vi "CmdExe.Text Log.vi"(7 "PrevLog":string, 8 "Rtn":i32, 9 "StdErr":string, 10 "StdOut":string, 11 "Cmd":string) -> (3 "CmdLog":string)   [LabVIEW 2019]
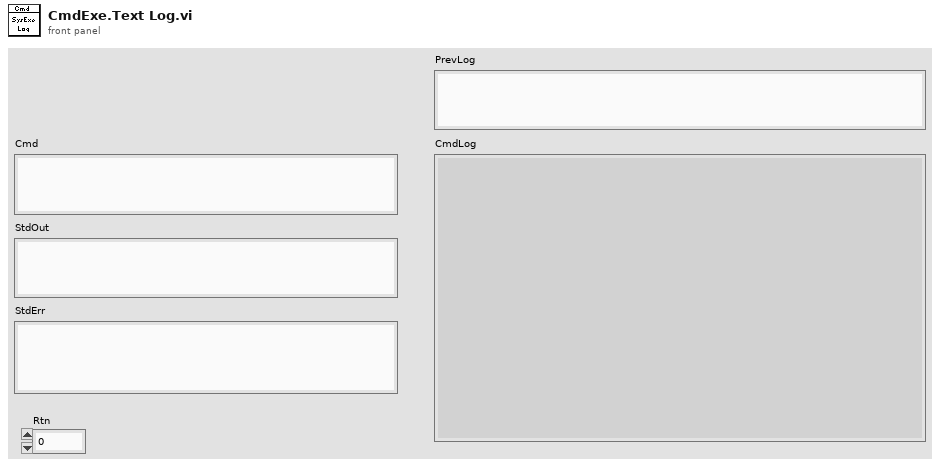
[diagram p1: front panel]
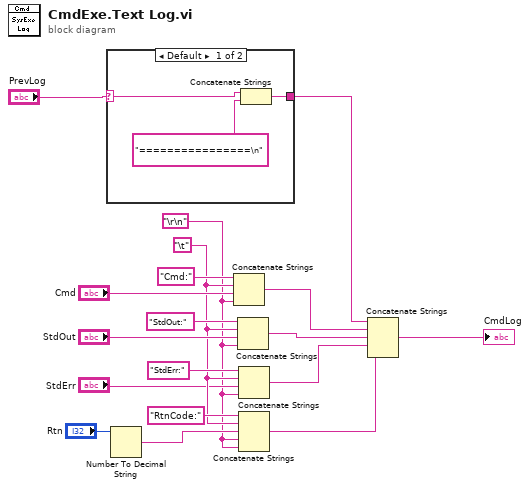
[diagram p0: block diagram]
diagram:
  w3 = "\r\n"
  w12 = "\t"
  n1 = case shown="Default" "PrevLog" {
    selector: "PrevLog" -> [w20 w22]
    tunnel: [w21 w22] -> w1
    frame Default {
      n2 = Concatenate Strings(w20, "================\n") -> (w21:string)
    }
    frame "" {
    }
  }
  n3 = Number To Decimal String(number="Rtn") -> (decimal integer string=w5:string)  [unwired: 1 in]
  n4 = Concatenate Strings("Cmd:", w12, "Cmd", w3) -> (w11:string)
  n5 = Concatenate Strings("StdOut:", w12, "StdOut", w3) -> (w10:string)
  n6 = Concatenate Strings("StdErr:", w12, "StdErr", w3) -> (w9:string)
  n7 = Concatenate Strings("RtnCode:", w12, w5, w3, w3) -> (w8:string)
  n8 = Concatenate Strings(w1, w11, w10, w9, w8) -> (→"CmdLog":string)
